vi "_Animate to Size & Position.vi"(5 "Delay mS":u32, 7 "Steps":i32, 8 "Callback Owner":refnum<class>, 9 "Done Callback":refnum<vi>, 10 "Dest Bounds":T1, 11 "VI Refnum":refnum<vi>) -> ()   [LabVIEW 2020, in "PicoG-Processor.lvlib"]
uses:
  PicoG-Processor.lvlib
  <vilib>/Utility/miscctls.llb/LVRectTypeDef.ctl
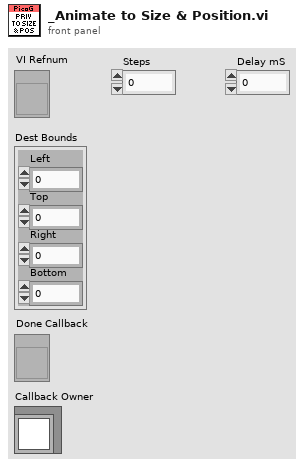
[diagram p1: front panel]
types:
  T1 = typedef "LVRectTypeDef.ctl" = cluster{"Left":i16, "Top":i16, "Right":i16, "Bottom":i16}
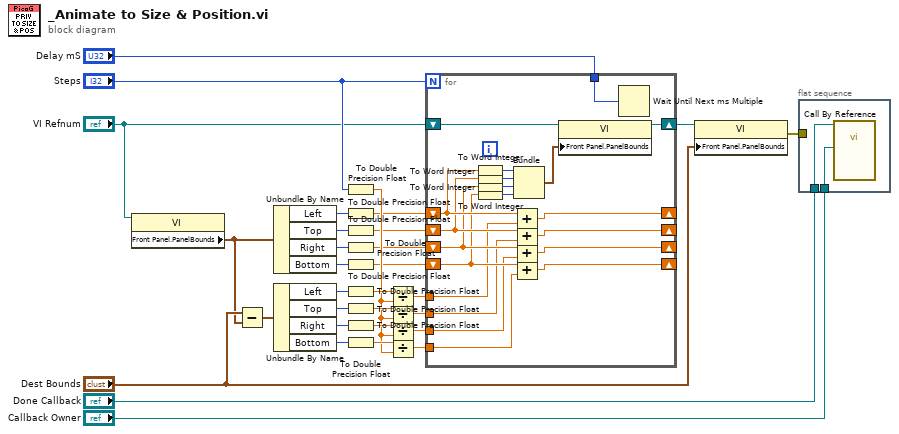
[diagram p0: block diagram]
diagram:
  n1 = property class="VI"(reference="VI Refnum") -> ("Front Panel.PanelBounds"=w4:T1)  [unwired: 1 in, 2 out]
  n2 = Subtract(x="Dest Bounds", y=w4) -> (x-y=w30:T1)
  n3 = Unbundle By Name(w4) -> ("Left"=w22:i16, "Top"=w23:i16, "Right"=w25:i16, "Bottom"=w24:i16)
  n4 = Unbundle By Name(w30) -> ("Left"=w29:i16, "Top"=w28:i16, "Right"=w26:i16, "Bottom"=w27:i16)
  n5 = To Double Precision Float(number="Steps") -> (double precision float=w17:dbl)
  n6 = To Double Precision Float(number=w22) -> (double precision float=w9:dbl)
  n7 = To Double Precision Float(number=w23) -> (double precision float=w10:dbl)
  n8 = To Double Precision Float(number=w25) -> (double precision float=w11:dbl)
  n9 = To Double Precision Float(number=w24) -> (double precision float=w12:dbl)
  n10 = To Double Precision Float(number=w29) -> (double precision float=w21:dbl)
  n11 = To Double Precision Float(number=w28) -> (double precision float=w20:dbl)
  n12 = To Double Precision Float(number=w26) -> (double precision float=w18:dbl)
  n13 = To Double Precision Float(number=w27) -> (double precision float=w19:dbl)
  n14 = Divide(x=w21, y=w17) -> (x/y=w16:dbl)
  n15 = Divide(x=w20, y=w17) -> (x/y=w15:dbl)
  n16 = Divide(x=w18, y=w17) -> (x/y=w14:dbl)
  n17 = Divide(x=w19, y=w17) -> (x/y=w13:dbl)
  n18 = for {
    N: "Steps" -> [_]
    shift-right: [w37] -> _
    shift-left: w9 -> [w45]
    shift-right: [w36] -> _
    shift-left: w10 -> [w44]
    shift-right: [w35] -> _
    shift-left: w11 -> [w43]
    shift-right: [w34] -> _
    shift-left: w12 -> [w42]
    tunnel: w16 -> [w38]
    tunnel: w15 -> [w39]
    tunnel: w14 -> [w40]
    tunnel: w13 -> [w41]
    shift-right: [w33] -> w7
    shift-left: "VI Refnum" -> [w46]
    tunnel: "Delay mS" -> [w32]
    n19 = To Word Integer(number=w45) -> (16bit integer=w51:i16)
    n20 = To Word Integer(number=w44) -> (16bit integer=w50:i16)
    n21 = To Word Integer(number=w43) -> (16bit integer=w49:i16)
    n22 = To Word Integer(number=w42) -> (16bit integer=w48:i16)
    n23 = Add(x=w45, y=w38) -> (x+y=w37:dbl)
    n24 = Add(x=w44, y=w39) -> (x+y=w36:dbl)
    n25 = Add(x=w43, y=w40) -> (x+y=w35:dbl)
    n26 = Add(x=w42, y=w41) -> (x+y=w34:dbl)
    n27 = Bundle(w51, w50, w49, w48) -> (w47:cluster{i16, i16, i16, i16})  [unwired: 1 in]
    n28 = property class="VI"(reference=w46, "Front Panel.PanelBounds"=w47) -> (reference out=w33:refnum<vi>)  [unwired: 1 in, 1 out]
    n29 = Wait Until Next ms Multiple(millisecond multiple=w32) -> ()  [unwired: 1 out]
  }
  n30 = property class="VI"(reference=w7, "Front Panel.PanelBounds"="Dest Bounds") -> (error out=w1:errorcluster)  [unwired: 1 in, 1 out]
  n31 = flat-sequence {
    tunnel: "Done Callback" -> [w53]
    tunnel: "Callback Owner" -> [w52]
    tunnel: w1 -> [_]
    frame #0 {
      n32 = call-by-ref "?"(reference=w53, "Owner"=w52) -> ()  [unwired: 12 in, 2 out]
    }
  }
